vi "tsapp_transmit_header_and_receive_msg.vi"(5 "ATimeoutMs":i32, 6 "ADLC":u8, 7 "错误输入（无错误）":errorcluster, 8 "AIdentifier":u8 format="%x", 9 "AChn":i32, 10 "Path":path) -> (0 "错误输出":errorcluster, 1 "return":i32, 2 "ALINData":T1, 3 "Path output":path)   [LabVIEW 2014]
doc: "Function Introduction :\nLIN master node: sends the header of LIN messages and receives LIN message data replied by slave nodes.\nCall location :\nThis function is used for the master node to send LIN message headers and receive data replies from the slave nodes.\ninput parameter :\nAChn: Channel\nAIdentifier: Message ID ADLC: Direct length of data to be received\nALINData: LIN message used to store received data</param>\nATimeoutMs: Receive wait timeout, if exceeded, receive fails\nReturn value :\n==0: Received successfully\nOther values: Received failed"
uses:
  Typedef/TLibLIN.ctl
panel:
  in  "TLIBLIN":T1
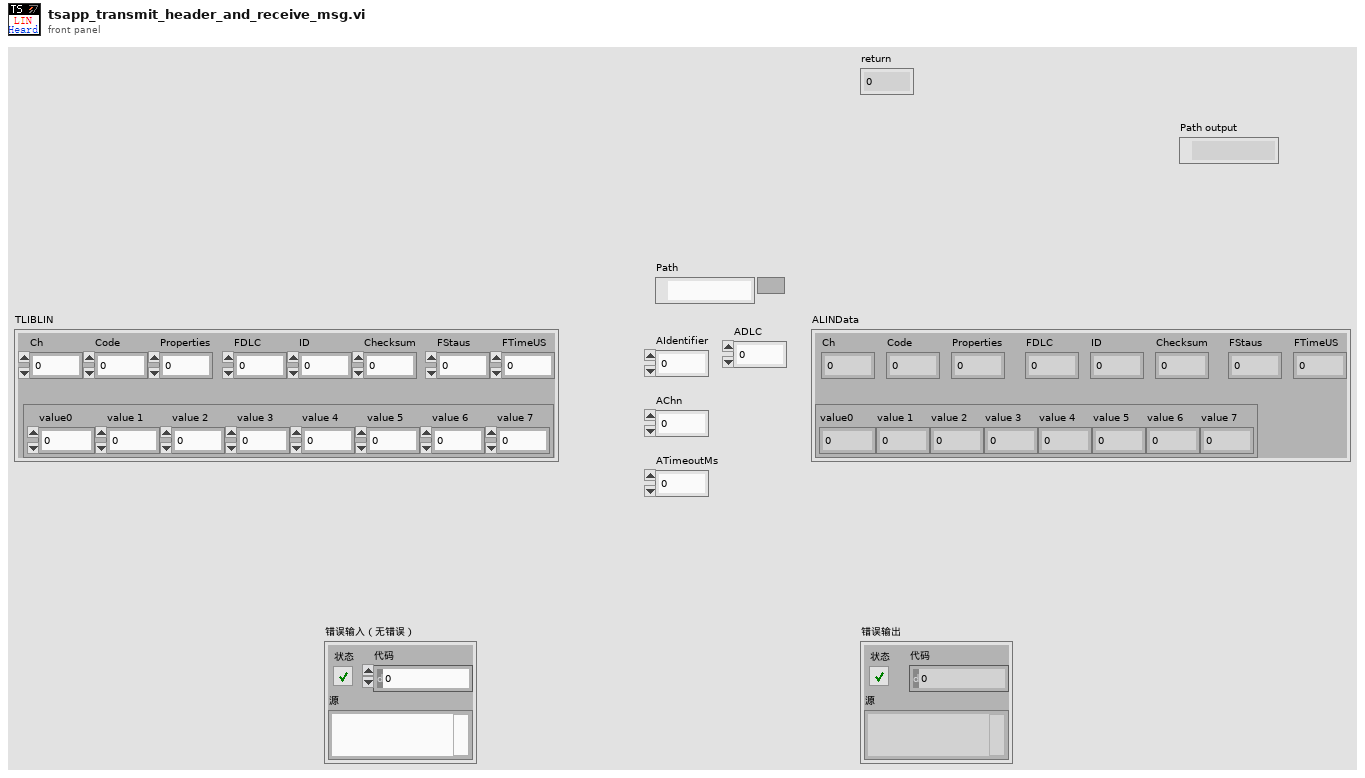
[diagram p1: front panel]
types:
  T1 = typedef "TLibLIN.ctl" = cluster{"Ch":u8, "Code":u8, "Properties":u8, "FDLC":u8, "ID":u8, "Checksum":u8, "FStaus":u8, "FTimeUS":u64, "FDatas":cluster{"value0":u8, "value 1":u8, "value 2":u8, "value 3":u8, "value 4":u8, "value 5":u8, "value 6":u8, "value 7":u8}}
  T2 = cluster{"value0":u8, "value 1":u8, "value 2":u8, "value 3":u8, "value 4":u8, "value 5":u8, "value 6":u8, "value 7":u8}
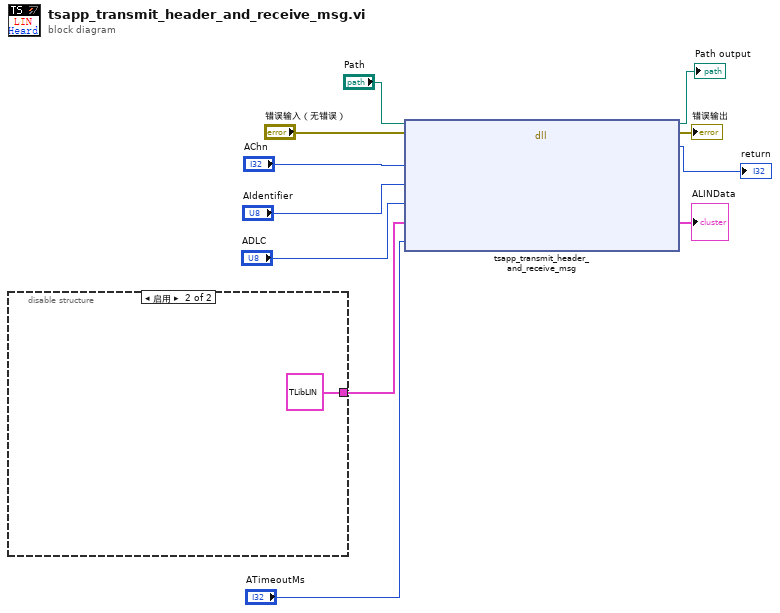
[diagram p0: block diagram]
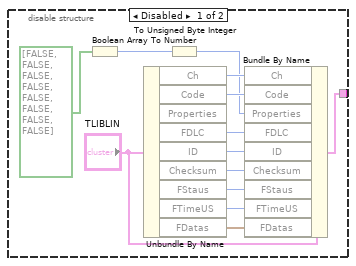
[diagram p2: hidden frame]
diagram:
  n1 = disable-structure shown="启用" {
    disable-tunnel: [w14 T1 {"Ch"=0, "Code"=0, "Properties"=0, "FDLC"=0, "ID"=0, "Checksum"=0, "FStaus"=0, "FTimeUS"=0, "FDatas"={"value0"=0, "value 1"=0, "value 2"=0, "value 3"=0, "value 4"=0, "value 5"=0, "value 6"=0, "value 7"=0}} ("TLIBLIN")] -> w8
    frame Disabled {
      n2 = Boolean Array To Number(Boolean array=bool[] [FALSE, FALSE, FALSE, FALSE, FALSE, FALSE, FALSE, FALSE]) -> (number=w17:u32)
      n3 = Unbundle By Name("TLIBLIN") -> ("Ch"=w24:u8, "Code"=w23:u8, "FDLC"=w22:u8, "ID"=w21:u8, "Checksum"=w20:u8, "FStaus"=w19:u8, "FTimeUS"=w18:u64, "FDatas"=w13:T2)  [unwired: 1 out]
      n4 = To Unsigned Byte Integer(number=w17) -> (unsigned 8bit integer=w15:u8)
      n5 = Bundle By Name(cluster="TLIBLIN", "Ch"=w24, "Code"=w23, "Properties"=w15, "FDLC"=w22, "ID"=w21, "Checksum"=w20, "FStaus"=w19, "FTimeUS"=w18, "FDatas"=w13) -> (w14:T1)
    }
    frame Enabled {
    }
  }
  n6 = dll-call lib="PTH2@abs EDemo同星TSCAN_V1.4_20220301ConfigTSMaster.dll" fn="tsapp_transmit_header_and_receive_msg"(path in="Path", error in="错误输入（无错误）", "AChn"="AChn", "AIdentifier"="AIdentifier", "ADLC"="ADLC", "ALINData"=w8, "ATimeoutMs"="ATimeoutMs") -> (path out=→"Path output":path, error out=→"错误输出":errorcluster, "tsapp_transmit_header_and_receive_msg"=→"return":i32, "ALINData"=→"ALINData":T1)  [unwired: 5 in]
